vi "String_Test (SubVI).vi"(8 "error in":errorcluster, 11 "Process name in":string) -> (0 "error out":errorcluster, 3 "Process name out":string)   [LabVIEW 2013]
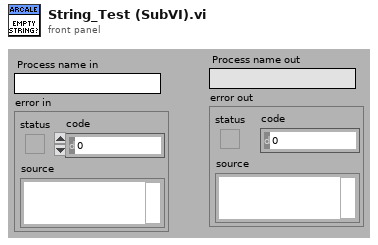
[diagram p1: front panel]
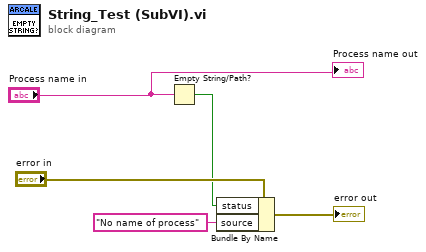
[diagram p0: block diagram]
diagram:
  n1 = Empty String/Path?(string/path="Process name in") -> (empty?=w4:bool)
  n2 = Bundle By Name(cluster="error in", "status"=w4, "source"="No name of process") -> (→"error out":errorcluster)
  "Process name out" <- "Process name in"
